vi "Module Not Synced--error.vi"() -> (0 "error out":errorcluster)   [LabVIEW 2020, in "Ophir Power Meter.lvlib"]
doc: "Outputs an error cluster containing a custom error code indicating the module events were unable to synchronize.\n_____\nBased on Delacor QMH Project Template 5.0.0.82."
uses:
  Ophir Power Meter.lvlib
  <vilib>/Utility/error.llb/Error Cluster From Error Code.vi
  <vilib>/ErrorRing/Error Ring.xnode
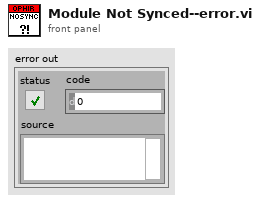
[diagram p1: front panel]
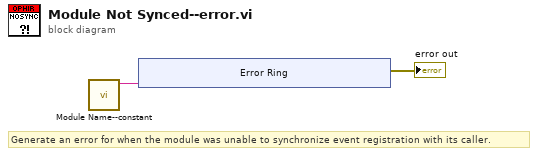
[diagram p0: block diagram]
diagram:
  # "Generate an error for when the module was unable to synchronize event registration with its caller."
  n1 = call "Module Name--constant.vi"() -> ("Module Name"=w1:string)  [unwired: 11 in]
  n2 = xnode "Error Ring"("parameter 0"=w1) -> ("error out"=→"error out":errorcluster)
